vi "Error Test Number Of Bits.vi"(6 "error text in":string, 7 "direction":T1, 8 "error in":errorcluster, 10 "number of bits":i32) -> (0 "error out":errorcluster)   [LabVIEW 2023]
uses:
  Direction.ctl
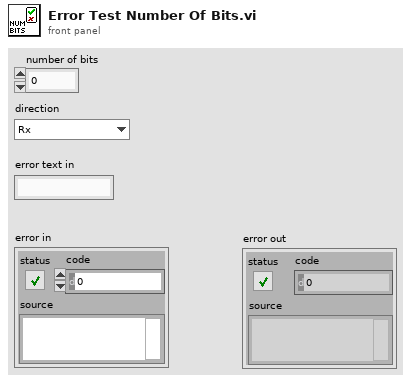
[diagram p1: front panel]
types:
  T1 = typedef "Direction.ctl" = enum16{"Rx", "Tx"}
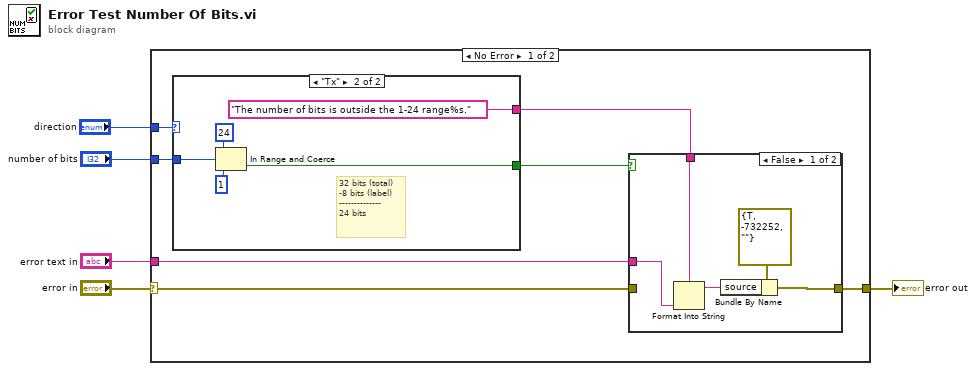
[diagram p0: block diagram]
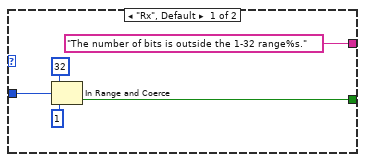
[diagram p3: hidden frame]
diagram:
  n1 = case shown="No Error" "error in" {
    selector: "error in" -> [w11 w29]
    tunnel: [w10 w29] -> w4
    tunnel: "number of bits" -> [w12 _]
    tunnel: "error text in" -> [w8 _]
    tunnel: "direction" -> [w7 _]
    frame No Error {
      n2 = case shown="\"Tx\"" w7 {
        tunnel: w12 -> [w23 w28]
        tunnel: [w20 w25] -> w9
        tunnel: ["The number of bits is outside the 1-32 range%s." ("source") "The number of bits is outside the 1-24 range%s." ("source")] -> w6
        frame "Rx", Default {
          n3 = In Range and Coerce(upper limit=32 ("lower limit"), x=w23, lower limit=1) -> (In Range?=w20:bool)  [unwired: 1 out]
        }
        frame "Tx" {
          # "32 bits (total)\n-8 bits (label)\n--------------\n24 bits"
          n4 = In Range and Coerce(upper limit=24 ("lower limit"), x=w28, lower limit=1) -> (In Range?=w25:bool)  [unwired: 1 out]
        }
      }
      n5 = case shown="False" w9 {
        tunnel: w11 -> [_ w18]
        tunnel: [w17 w18] -> w10
        tunnel: w8 -> [w16 _]
        tunnel: w6 -> [w14 _]
        frame False {
          n6 = Format Into String(format string=w14, w16) -> (resulting string=w15:string)  [unwired: 2 in, 1 out]
          n7 = Bundle By Name(cluster=errorcluster {"status"=TRUE, "code"=-732252, "source"=""} ("error constant"), "source"=w15) -> (w17:errorcluster)
        }
        frame True {
        }
      }
    }
    frame Error {
    }
  }
  "error out" <- w4
